vi "Pixel Scan Parameters AE.vi"(2 "Action":enum16{"Write", "Read"}(ring), 7 "Pixel Scan Parameters":T1={"Scan Start Pixel"=1, "Scan End Pixel"=1, "Pixel Start Value (-1 to 1)"=-0.5, "Pixel End Value (-1 to 1)"=0.5, "Number of Steps"=0.1}) -> (8 "Pixel Scan Parameters Out":T1={"Scan Start Pixel"=1, "Scan End Pixel"=1, "Pixel Start Value (-1 to 1)"=-0.5, "Pixel End Value (-1 to 1)"=0.5, "Number of Steps"=0.1})   [LabVIEW 2014]
uses:
  Controls/Pixel Scan Parameters.ctl
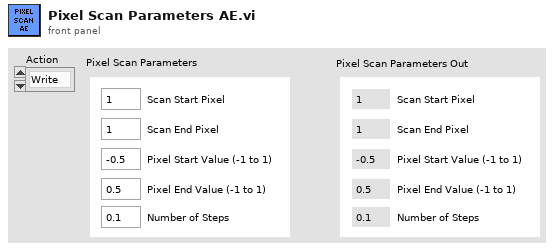
[diagram p1: front panel]
types:
  T1 = typedef "Pixel Scan Parameters.ctl" = cluster{"Scan Start Pixel":i32, "Scan End Pixel":i32, "Pixel Start Value (-1 to 1)":dbl, "Pixel End Value (-1 to 1)":dbl, "Number of Steps":dbl}
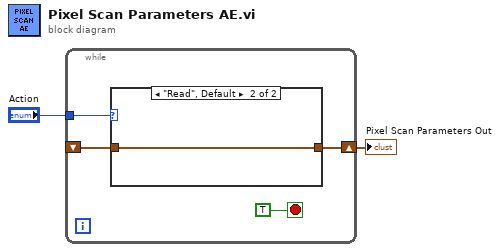
[diagram p0: block diagram]
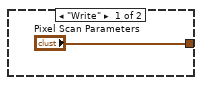
[diagram p2: hidden frame]
diagram:
  n1 = while {
    tunnel: "Action" -> [w5]
    shift-right: [w4] -> w1
    shift-left: _ -> [w3]
    stop <- TRUE stop-if-true
    n2 = case shown="\"Read\", Default" w5 {
      tunnel: ["Pixel Scan Parameters" w8] -> w4
      tunnel: w3 -> [_ w8]
      frame "Write" {
      }
      frame "Read", Default {
      }
    }
  }
  "Pixel Scan Parameters Out" <- w1
